vi "CC Convert DEC to String.vi"(8 "error in (no error)":errorcluster, 11 "DEC":dbl) -> (0 "error out":errorcluster, 2 "Declination":T1 {"Arc Sec" format="%0#2_6g"}, 3 "DEC String":string)   [LabVIEW 2024]
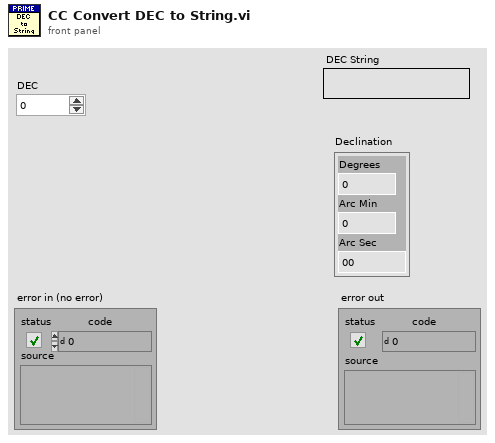
[diagram p1: front panel]
types:
  T1 = cluster{"Degrees":dbl, "Arc Min":dbl, "Arc Sec":dbl}
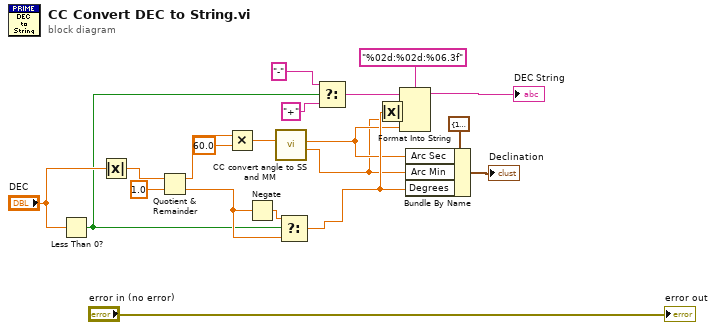
[diagram p0: block diagram]
diagram:
  n1 = Less Than 0?(x="DEC") -> (x < 0?=w5:bool)
  n2 = Absolute Value(x="DEC") -> (abs(x)=w13:dbl)
  n3 = Quotient & Remainder(x=w13, y=1.0) -> (x-y*floor(x/y)=w19:dbl, floor(x/y)=w11:dbl)
  n4 = Multiply(x=w19, y=60.0) -> (x*y=w8:dbl)
  n5 = Negate(x=w11) -> (-x=w12:dbl)
  n6 = call "CC convert angle to SS and MM.vi"("Angle"=w8) -> ("Minutes"=w6:dbl, "Seconds"=w7:dbl)  [unwired: 9 in]
  n7 = Select(t=w12, s=w5, f=w11) -> (s? t:f=w10:dbl)
  n8 = Select(t="-", s=w5, f="+") -> (s? t:f=w2:string)
  n9 = Absolute Value(x=w10) -> (abs(x)=w1:dbl)
  n10 = Format Into String(format string="%02d:%02d:%06.3f", initial string=w2, w1, w6, w7) -> (resulting string=→"DEC String":string)  [unwired: 1 in, 1 out]
  n11 = Bundle By Name(cluster=T1 {"Degrees"=10.0, "Arc Min"=2.0, "Arc Sec"=11.040000000001555} ("Declination"), "Arc Sec"=w7, "Arc Min"=w6, "Degrees"=w10) -> (→"Declination":T1)
  "error out" <- "error in (no error)"
